vi "Characters_to_string.vi"(1 "Characters to write":string, 2 "Label for characters":string) -> (0 "Output string":string)   [LabVIEW 2017]
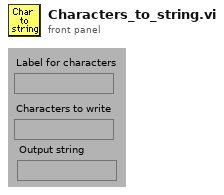
[diagram p1: front panel]
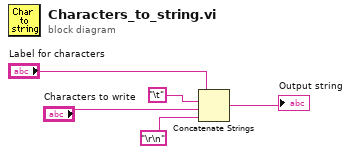
[diagram p0: block diagram]
diagram:
  n1 = Concatenate Strings("Label for characters", "\t", "Characters to write", "\r\n") -> (→"Output string":string)
